vi "FP behavior P-Wall.vi"(1 "Behavior\nVelocity":dbl=20.0, 2 "Activate?":bool=TRUE, 3 "IR Sensors":T1(array[cluster])) -> (0 "P-Wall Array":dbl[](array[numeric]))   [LabVIEW 2014]
doc: "This vi creates a array based upon the value of the PBow IR sensor reading."
uses:
  <vilib>/addons/control/pid/pid.llb/PID (DBL).vi
  <vilib>/addons/control/pid/NI_PID_pid.lvlib
panel:
  out "HPort Setpoint":dbl=40.0 format="%#_13g"
  out "Half-Port\nSensor":string
  out "Port Setpoint":dbl=40.0 format="%#_13g"
  out "steer":dbl format="%.2f"
  out "Port Side Sensor":string
  out "Waveform Graph":cluster{dbl, dbl, dbl[]}(graph)
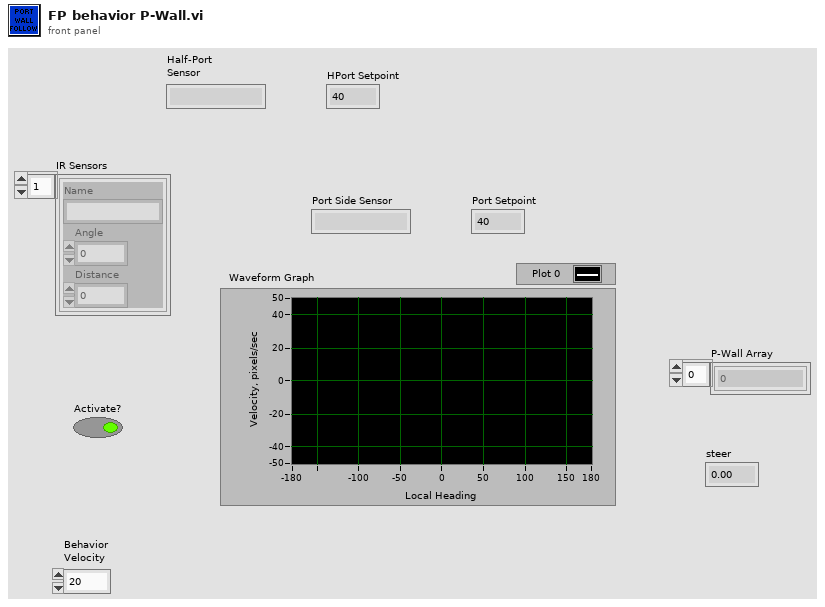
[diagram p1: front panel]
types:
  T1 = cluster{"Name":string, "Angle":dbl, "Distance":dbl}[]
  T2 = cluster{"proportional gain (Kc)":dbl, "integral time (Ti, min)":dbl, "derivative time (Td, min)":dbl}
  T3 = cluster{"Name":string, "Angle":dbl, "Distance":dbl}
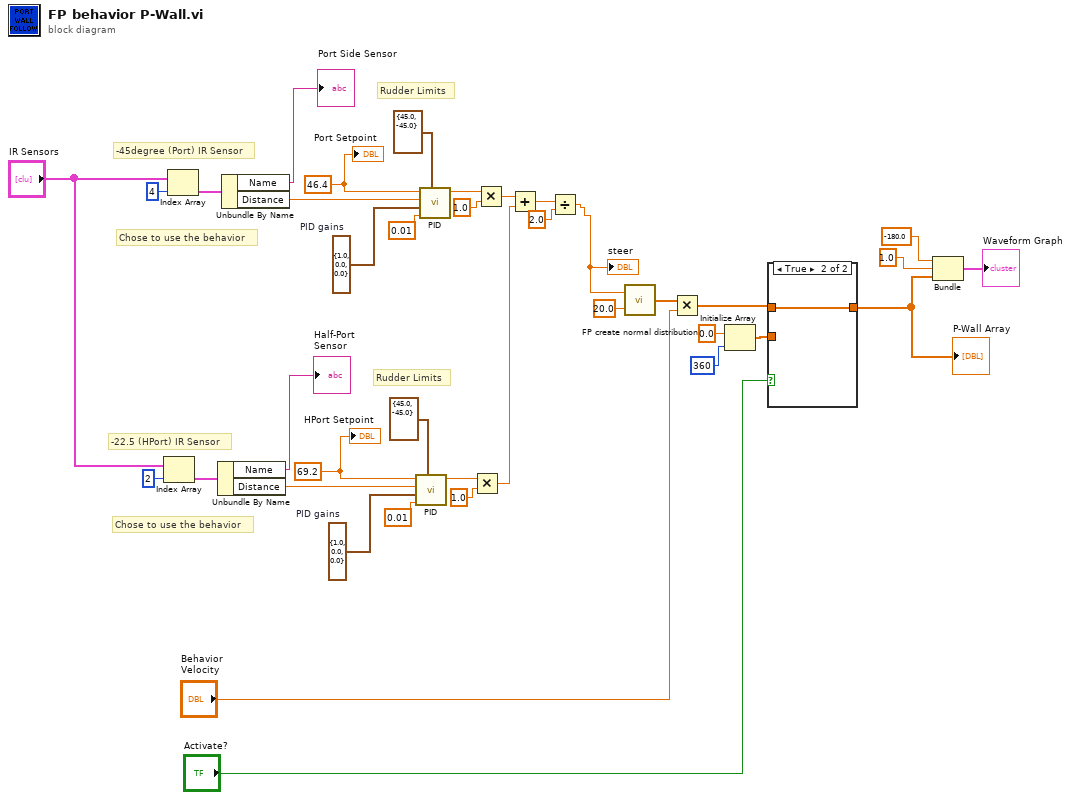
[diagram p0: block diagram]
diagram:
  w3 = 69.2 ("Port Setpoint")
  w4 = 46.4 ("Port Setpoint")
  w10 = T2 {"proportional gain (Kc)"=1.0, "integral time (Ti, min)"=0.0, "derivative time (Td, min)"=0.0}  # PID gains
  w23 = T2 {"proportional gain (Kc)"=1.0, "integral time (Ti, min)"=0.0, "derivative time (Td, min)"=0.0}  # PID gains
  # "-22.5 (HPort) IR Sensor"
  # "-45degree (Port) IR Sensor"
  # "Rudder Limits"
  # "Chose to use the behavior"
  # "Rudder Limits"
  # "Chose to use the behavior"
  n1 = Index Array(array="IR Sensors", index=2) -> (element=w16:T3)
  n2 = Index Array(array="IR Sensors", index=4) -> (element=w29:T3)
  n3 = Unbundle By Name(w16) -> ("Name"=→"Half-Port\nSensor":string, "Distance"=w9:dbl)
  n4 = Unbundle By Name(w29) -> ("Name"=→"Port Side Sensor":string, "Distance"=w22:dbl)
  n5 = call-poly <vilib>:"PID.vi"("output range"=cluster{"output high":dbl, "output low":dbl} {"output high"=45.0, "output low"=-45.0}, "dt (s)"=0.01, "PID gains"=w10, "process variable"=w9, "setpoint"=w3) -> ("output"=w13:dbl)  [unwired: 5 in, 1 out]
  n6 = call-poly <vilib>:"PID.vi"("output range"=cluster{"output high":dbl, "output low":dbl} {"output high"=45.0, "output low"=-45.0}, "dt (s)"=0.01, "PID gains"=w23, "process variable"=w22, "setpoint"=w4) -> ("output"=w26:dbl)  [unwired: 5 in, 1 out]
  n7 = Multiply(x=w13, y=1.0) -> (x*y=w7:dbl)
  n8 = Multiply(x=w26, y=1.0) -> (x*y=w2:dbl)
  n9 = Add(x=w2, y=w7) -> (x+y=w5:dbl)
  n10 = Divide(x=w5, y=2.0) -> (x/y=w1:dbl)
  "steer" <- w1
  n11 = call "FP create normal distribution.vi"("std (Normal)"=20.0, "mean"=w1) -> ("ACT array"=w21:dbl[])
  n12 = Multiply(x=w21, y="Behavior\nVelocity") -> (x*y=w20:dbl[])
  n13 = Initialize Array(0.0 ("element"), 360 ("dimension size")) -> (w32:dbl[])
  n14 = case shown="True" "Activate?" {
    tunnel: w32 -> [w39 _]
    tunnel: w20 -> [_ w40]
    tunnel: [w39 w40] -> w31
    frame False {
    }
    frame True {
    }
  }
  "P-Wall Array" <- w31
  n15 = Bundle(-180.0, 1.0, w31) -> (→"Waveform Graph":cluster{dbl, dbl, dbl[]})  [unwired: 1 in]
  "Port Setpoint" <- w4
  "HPort Setpoint" <- w3
